vi "test_programm_webcam.vi"() -> ()   [LabVIEW 2014]
uses:
  <vilib>/userdefined/High Color/IMAQdx.ctl
  <vilib>/vision/driver/NI_Vision_Acquisition_Software.lvlib
  <vilib>/vision/NI_Vision_Development_Module.lvlib
panel:
  in  "pattern2":bool
  in  "Pattern2 Farbe":u32(colorbox)=16711680
  in  "x":i32
  in  "y":i32
  out "Pattern1 2":T1(plugin-control)
  in  "Template File Path (Pattern Matching 2)":path=path "C:/Users/Kroll/Desktop/Test_04012016/Pattern/pattern_1412.png"
  out "date/time string":string
  in  "file path (dialog if empty)":path=path "I:/123.txt"
  in  "Länge der Spur":i32=50
  out "Pattern1":T1(plugin-control)
  in  "Template File Path (Pattern Matching 1)":path=path "C:/Users/Kroll/Desktop/Test_04012016/Pattern/pattern_1412.png"
  out "Image 2":T1(plugin-control)
  in  "Programm anhalten":bool
  in  "Parameters Pattern":T2={"Number of Matches Requested"=1, "Minimum Match Score"=800.0, "Angle Ranges"=[{"Start Angle"=-180.0, "End Angle"=180.0}, {"Start Angle"=0.0, "End Angle"=360.0}]}
  in  "Mittelpunktgröße":sgl
  in  "millisecond multiple":u32
  out "Processed Frames/s":dbl
  in  "Länge des Pfeils":sgl=80.0
  out "Acquired Frames/s":dbl
  in  "pattern1":bool
  in  "Pattern1 Farbe":u32(colorbox)=16711680
  in  "x":i32
  in  "y":i32
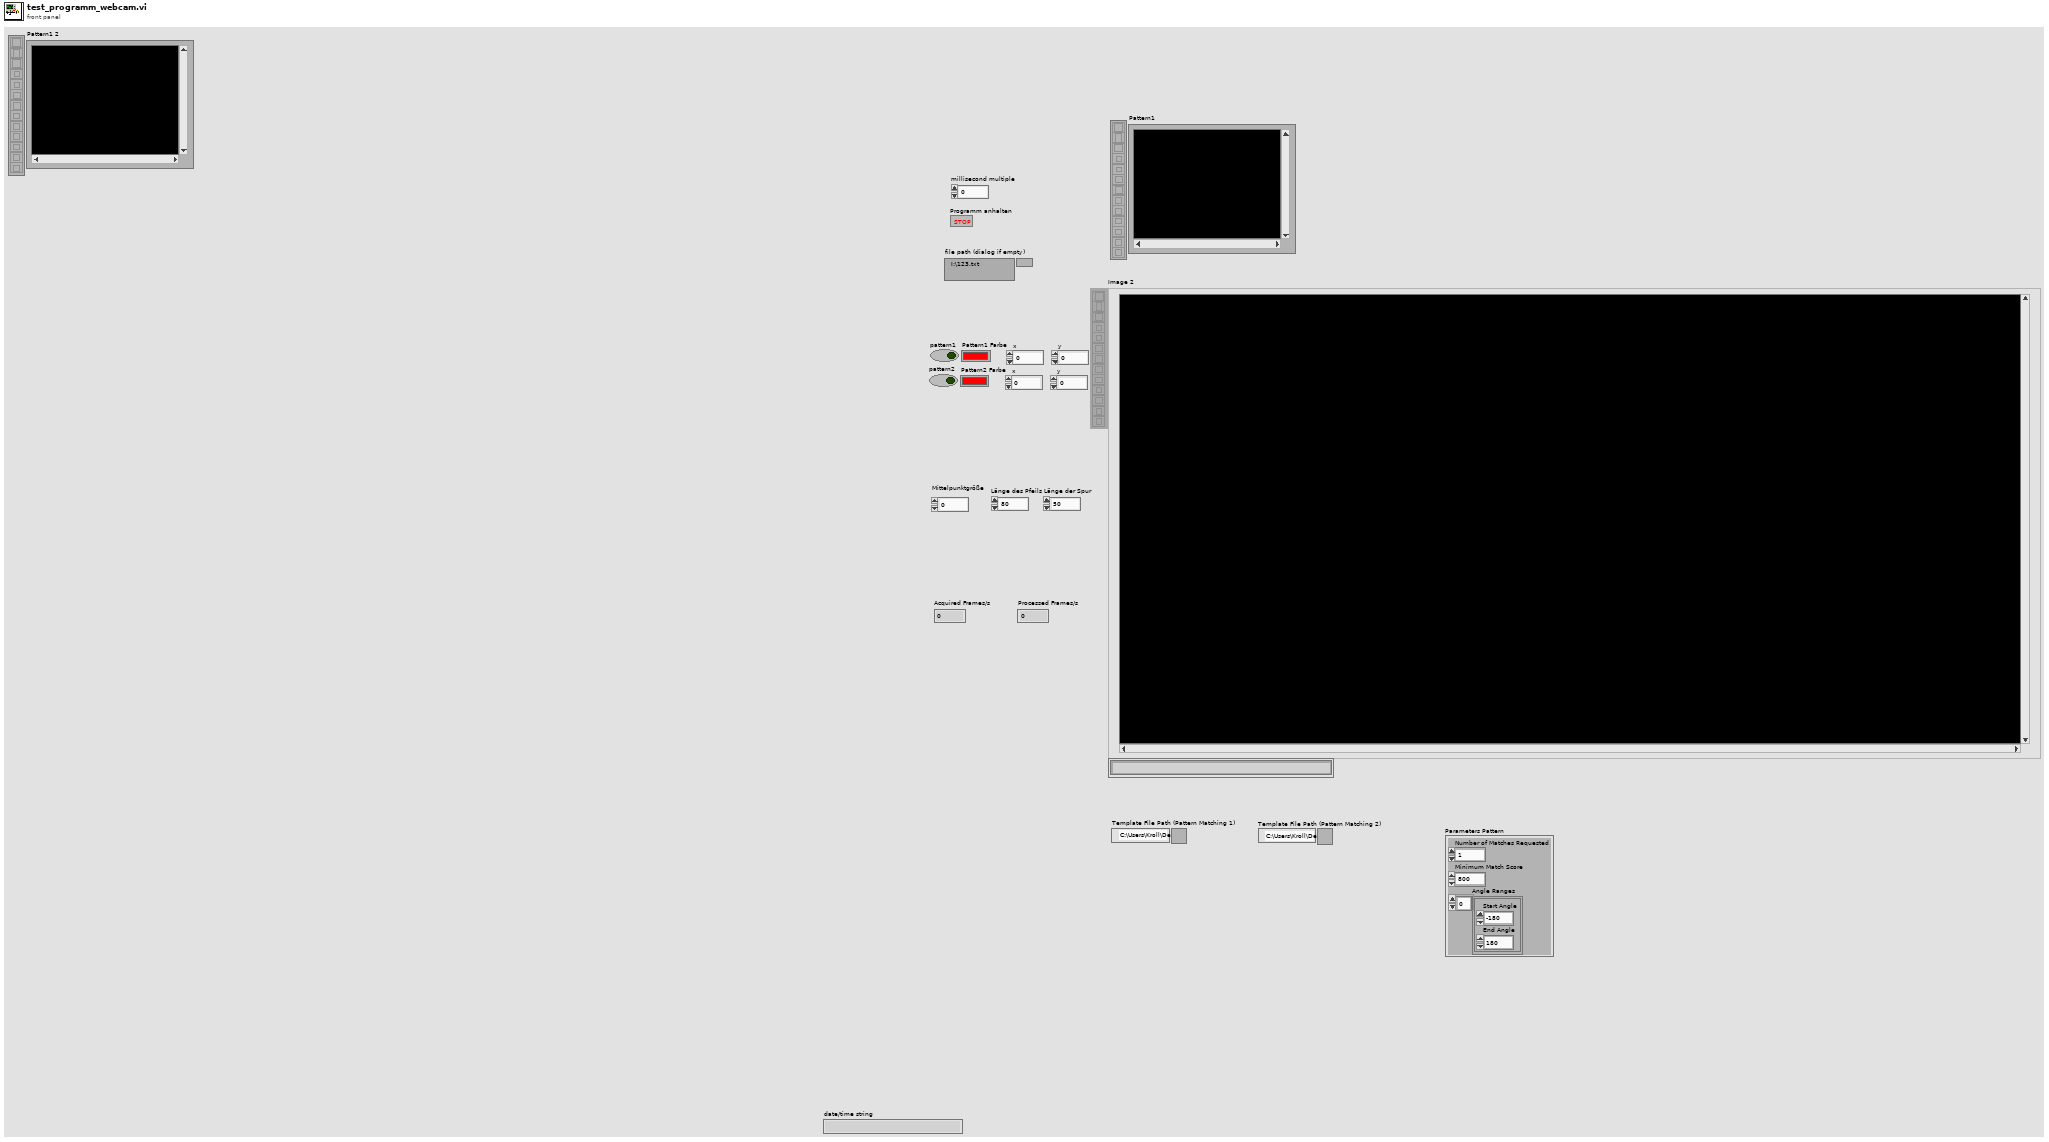
[diagram p1: front panel]
types:
  T1 = typedef "IMAQ Image.ctl" = refnum<image>
  T2 = cluster{"Number of Matches Requested":i32, "Minimum Match Score":sgl, "Angle Ranges":cluster{"Start Angle":sgl, "End Angle":sgl}[]}
  T3 = cluster{"Number of Histogram Bins":i32, "Blending Parameter (%)":dbl, "Maximum Iterations":i32}
  T4 = typedef "Image Type" = u32
  T5 = enum16{"open", "replace", "create", "open or create", "replace or create", "replace or create with confirmation"}
  T6 = typedef "IMAQdx.ctl" = refnum<k21>
  T7 = typedef "IMAQ Object Tracking Session.ctl" = refnum<k20>
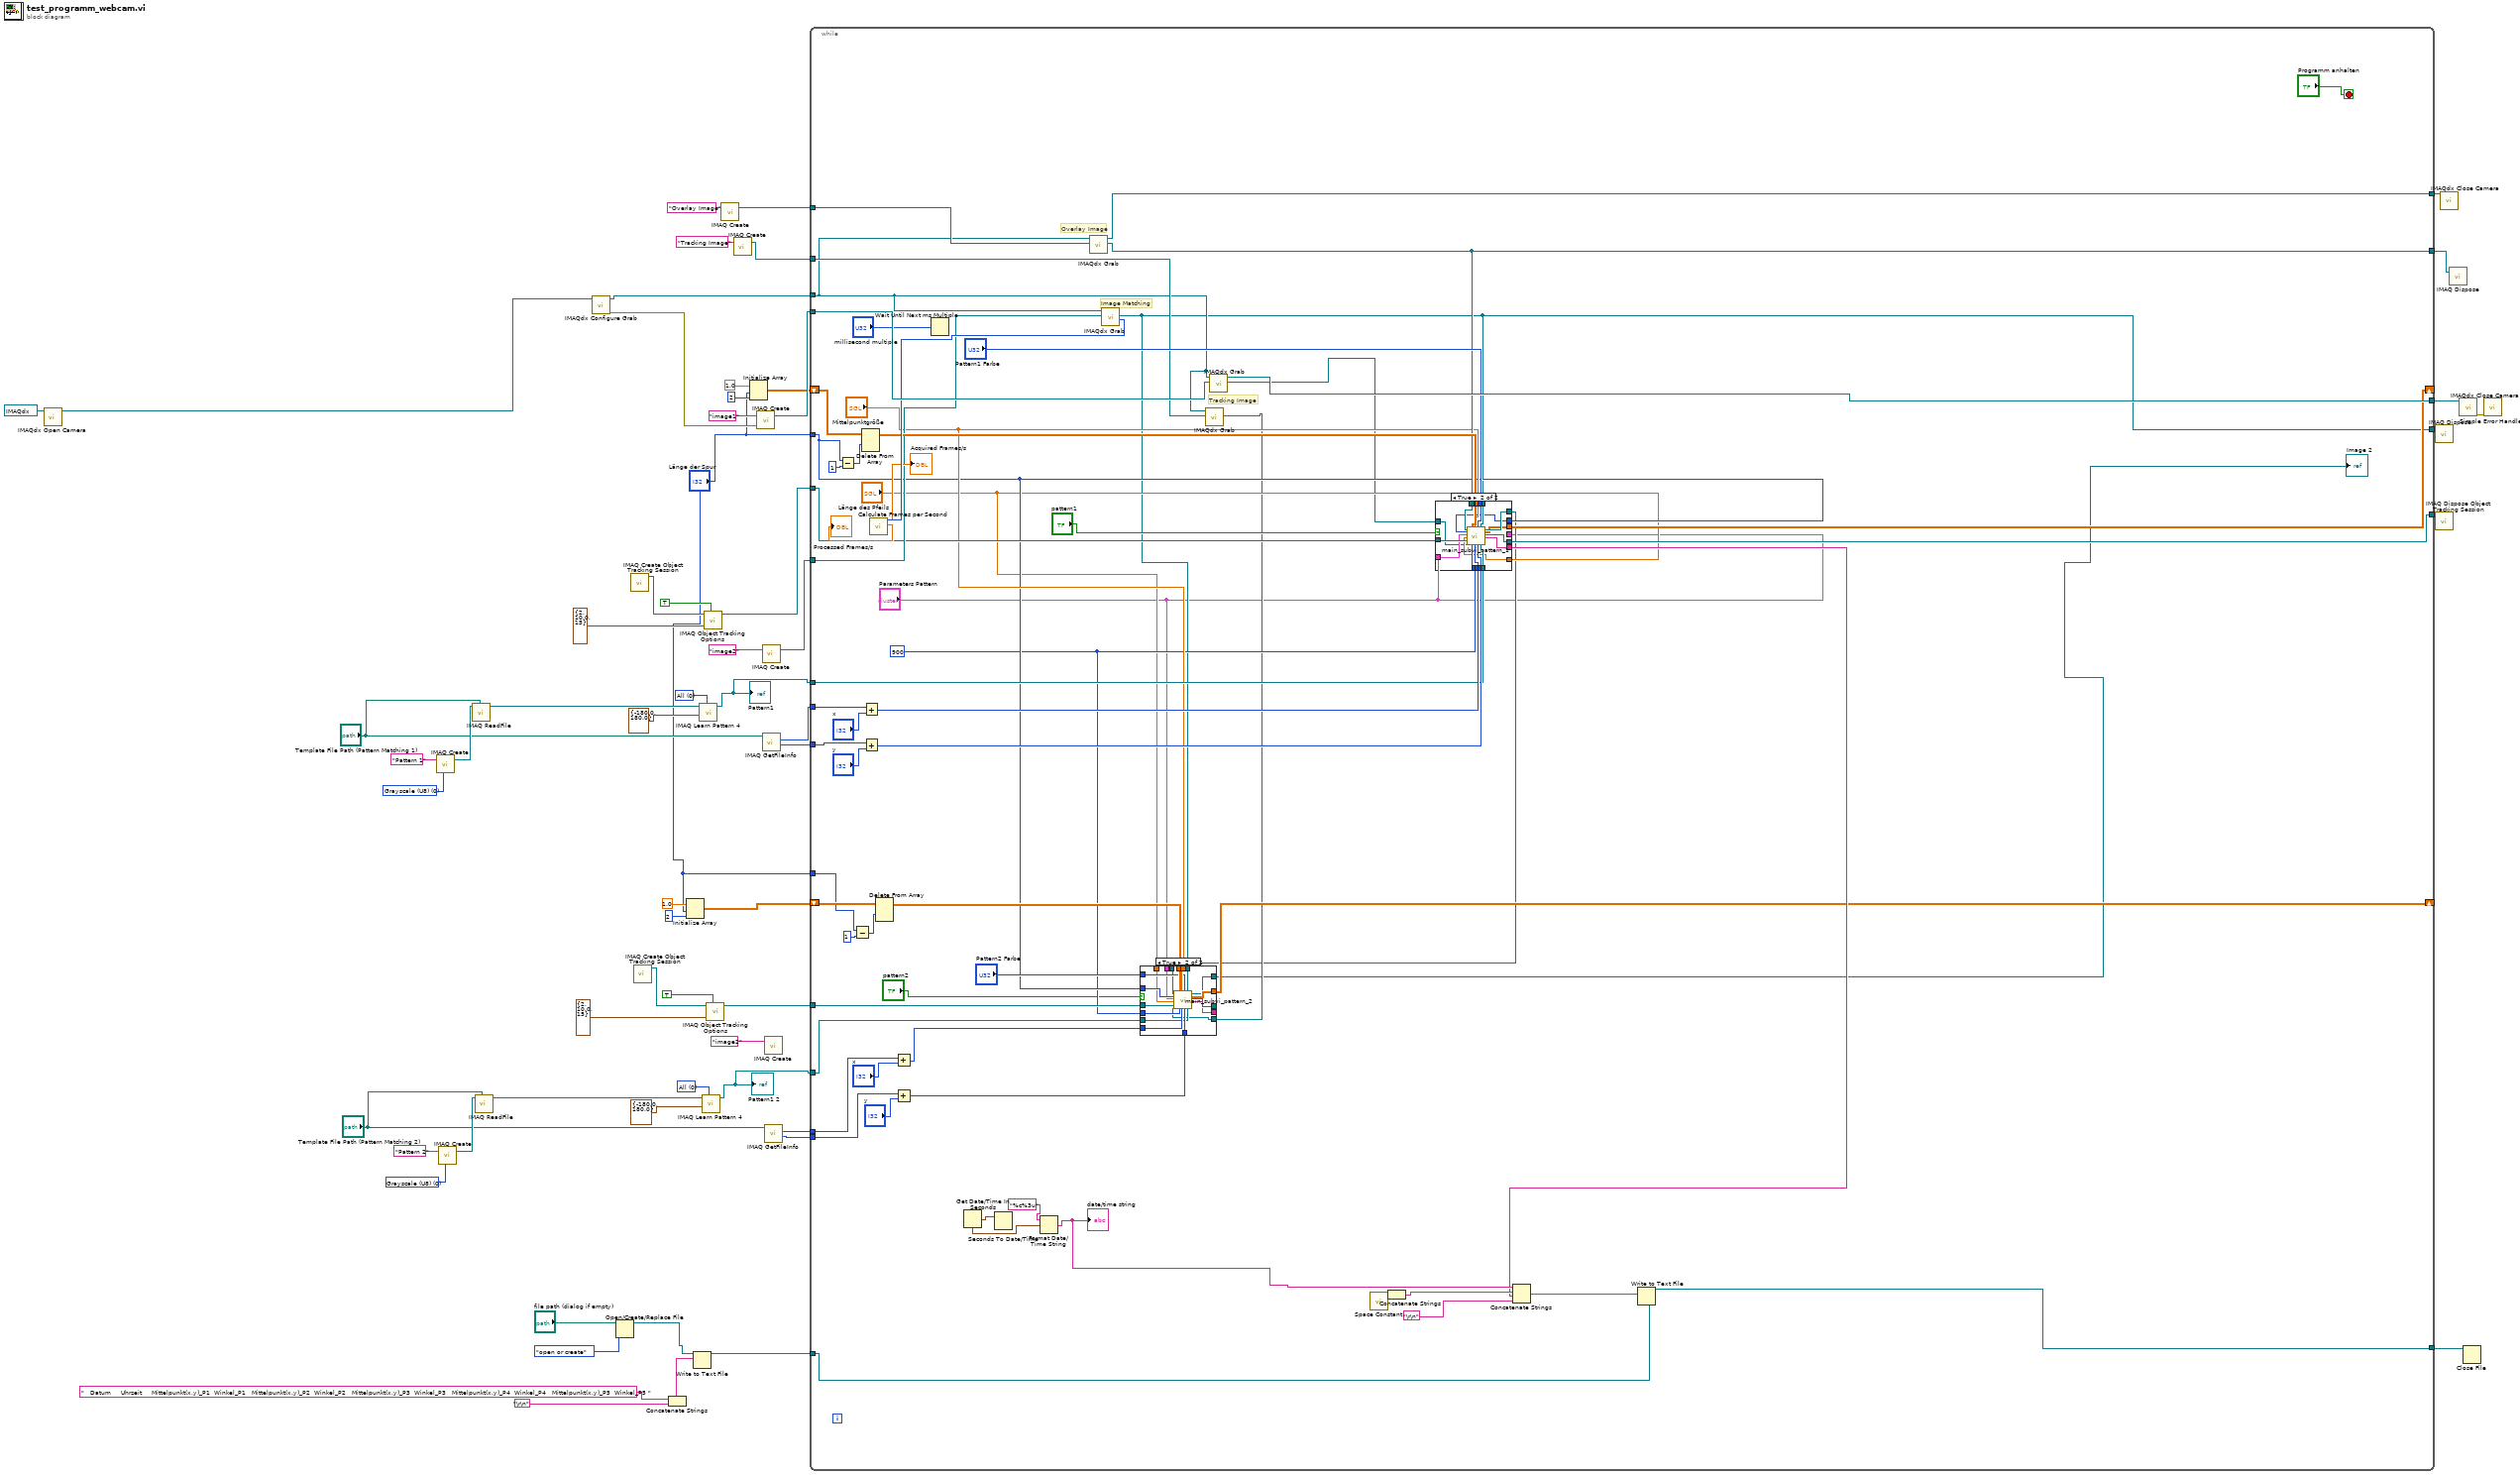
[diagram p0: block diagram]
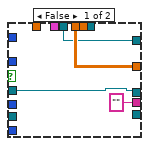
[diagram p2: hidden frame]
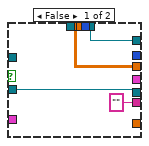
[diagram p3: hidden frame]
diagram:
  w16 = T4 0 items=["Grayscale (U8)", "Grayscale (I16)", "Grayscale (SGL)", "Complex (CSG)", "RGB (U32)", "HSL (U32)", "RGB (U64)", "Grayscale (U16)"] ("Image Type")
  w20 = 0 items=["All", "Low Discrepancy Sampling", "Grayscale Value Pyramid", "Gradients Pyramid"] ("Algorithm")
  w44 = T4 0 items=["Grayscale (U8)", "Grayscale (I16)", "Grayscale (SGL)", "Complex (CSG)", "RGB (U32)", "HSL (U32)", "RGB (U64)", "Grayscale (U16)"] ("Image Type")
  w48 = 0 items=["All", "Low Discrepancy Sampling", "Grayscale Value Pyramid", "Gradients Pyramid"] ("Algorithm")
  n1 = call <vilib>:"IMAQdx Open Camera.vi"("Session In"=T6 "cam4") -> ("Session Out"=w31:T6)  [unwired: 9 in, 1 out]
  n2 = call "IMAQ Create"("Image Name"="Pattern 1", "Image Type"=w44) -> ("New Image"=w45:T1)  [unwired: 3 in, 1 out]
  n3 = call "IMAQ Create"("Image Name"="Pattern 2", "Image Type"=w16) -> ("New Image"=w17:T1)  [unwired: 3 in, 1 out]
  n4 = call "IMAQ ReadFile"("File Path"="Template File Path (Pattern Matching 1)", "Image"=w45) -> ("Image Out"=w41:T1)  [unwired: 5 in, 4 out]
  n5 = call "IMAQ ReadFile"("File Path"="Template File Path (Pattern Matching 2)", "Image"=w17) -> ("Image Out"=w14:T1)  [unwired: 5 in, 4 out]
  n6 = call <vilib>:"IMAQdx Configure Grab.vi"("Session In"=w31) -> ("error out"=w62:errorcluster, "Session Out"=w60:T6)  [unwired: 9 in]
  n7 = Open/Create/Replace File(file path (use dialog)="file path (dialog if empty)", operation (0:open)=T5."open or create") -> (refnum out=w28:refnum<file>)  [unwired: 4 in, 2 out]
  n8 = call "IMAQ Create Object Tracking Session"() -> ("Object Tracking Session"=w40:T7)  [unwired: 1 in, 10 out]
  n9 = call "IMAQ Create Object Tracking Session"() -> ("Object Tracking Session"=w13:T7)  [unwired: 1 in, 10 out]
  n10 = Concatenate Strings("   Datum     Uhrzeit     Mittelpunkt(x,y)_P1  Winkel_P1   Mittelpunkt(x,y)_P2  Winkel_P2   Mittelpunkt(x,y)_P3  Winkel_P3   Mittelpunkt(x,y)_P4  Winkel_P4   Mittelpunkt(x,y)_P5  Winkel_P5 " ("string"), "\r\n") -> (w26:string)
  n11 = Initialize Array "Initialize Array"(1.0 ("element"), "Länge der Spur", 2 ("dimension size")) -> (w4:dbl[][])
  n12 = Write to Text File(file (use dialog)=w28, text=w26) -> (refnum out=w24:refnum<file>)  [unwired: 2 in, 2 out]
  n13 = call "IMAQ Learn Pattern 4"("Algorithm"=w48, "Angle Range"=cluster{"Start Angle":sgl, "End Angle":sgl} {"Start Angle"=-180.0, "End Angle"=180.0}, "Image"=w41) -> ("Template Image Out"=w42:T1)  [unwired: 6 in, 2 out]
  "Pattern1" <- w42
  n14 = call "IMAQ Learn Pattern 4"("Algorithm"=w20, "Angle Range"=cluster{"Start Angle":sgl, "End Angle":sgl} {"Start Angle"=-180.0, "End Angle"=180.0}, "Image"=w14) -> ("Template Image Out"=w9:T1)  [unwired: 6 in, 2 out]
  "Pattern1 2" <- w9
  n15 = call-poly "IMAQ Object Tracking Options"("Get/Set (Get)"=TRUE, "Mean Shift Options in"=T3 {"Number of Histogram Bins"=2, "Blending Parameter (%)"=10.0, "Maximum Iterations"=15}, "Object Tracking Session In"=w40) -> ("Object Tracking Session Out"=w39:T7)  [unwired: 6 in, 2 out]
  n16 = call-poly "IMAQ Object Tracking Options"("Get/Set (Get)"=TRUE, "Mean Shift Options in"=T3 {"Number of Histogram Bins"=2, "Blending Parameter (%)"=10.0, "Maximum Iterations"=15}, "Object Tracking Session In"=w13) -> ("Object Tracking Session Out"=w10:T7)  [unwired: 6 in, 2 out]
  n17 = call "IMAQ Create"("Image Name"="Overlay Image") -> ("New Image"=w35:T1)  [unwired: 4 in, 1 out]
  n18 = call "IMAQ Create"("Image Name"="Tracking Image") -> ("New Image"=w1:T1)  [unwired: 4 in, 1 out]
  n19 = Initialize Array "Initialize Array"(1.0 ("element"), "Länge der Spur", 2 ("dimension size")) -> (w50:dbl[][])
  n20 = call "IMAQ Create"("Image Name"="image1", "error in (no error)"=w62) -> ("New Image"=w59:T1)  [unwired: 3 in, 1 out]
  n21 = call "IMAQ Create"("Image Name"="image2") -> ("New Image"=w55:T1)  [unwired: 4 in, 1 out]
  n22 = call "IMAQ GetFileInfo"("File Path"="Template File Path (Pattern Matching 1)") -> ("Y Resolution"=w52:i32, "X Resolution"=w53:i32)  [unwired: 4 in, 5 out]
  n23 = call "IMAQ Create"("Image Name"="image2") -> ()  [unwired: 4 in, 2 out]
  n24 = call "IMAQ GetFileInfo"("File Path"="Template File Path (Pattern Matching 2)") -> ("Y Resolution"=w7:i32, "X Resolution"=w8:i32)  [unwired: 4 in, 5 out]
  n25 = while {
    tunnel: w60 -> [w68]
    tunnel: w59 -> [w126]
    tunnel: [w127] -> w57
    tunnel: [w64] -> w54
    tunnel: w55 -> [w112]
    tunnel: w53 -> [w113]
    tunnel: w52 -> [w114]
    shift-right: [w105] -> _
    shift-left: w50 -> [w121]
    tunnel: "Länge der Spur" -> [w80]
    tunnel: w42 -> [w102]
    tunnel: w39 -> [w106]
    tunnel: [w111] -> w37
    tunnel: w35 -> [w108]
    tunnel: [w103] -> w34
    tunnel: [w107] -> w33
    tunnel: w24 -> [w99]
    tunnel: [w95] -> w23
    tunnel: w10 -> [w79]
    tunnel: w9 -> [w75]
    tunnel: w8 -> [w90]
    tunnel: w7 -> [w89]
    shift-right: [w83] -> _
    shift-left: w4 -> [w86]
    tunnel: "Länge der Spur" -> [w85]
    tunnel: w1 -> [w69]
    stop <- "Programm anhalten" stop-if-true
    w78 = 900 ("Minimum Score")
    # "Overlay Image"
    # "Image Matching"
    # "Tracking Image"
    n26 = Subtract(x=w80, y=1) -> (x-y=w118:i32)
    n27 = Subtract(x=w85, y=1) -> (x-y=w87:i32)
    n28 = Delete From Array "Delete From Array"(array=w121, index (row)=w118) -> (array with subset deleted=w120:dbl[][])  [unwired: 2 in, 1 out]
    n29 = Add(x=w113, y="x") -> (x+y=w110:i32)
    n30 = Add(x=w114, y="y") -> (x+y=w109:i32)
    n31 = Delete From Array "Delete From Array"(array=w86, index (row)=w87) -> (array with subset deleted=w84:dbl[][])  [unwired: 2 in, 1 out]
    n32 = Add(x=w90, y="x") -> (x+y=w76:i32)
    n33 = Add(x=w89, y="y") -> (x+y=w77:i32)
    n34 = Wait Until Next ms Multiple(millisecond multiple="millisecond multiple") -> ()  [unwired: 1 out]
    n35 = Get Date/Time In Seconds() -> (seconds since 1Jan1904=w98:timestamp)
    n36 = Seconds To Date/Time(time stamp (now)=w98) -> ()  [unwired: 1 in, 1 out]
    n37 = Format Date/Time String(time format string (%c)="%c%3u", seconds (now)=w98) -> (date/time string=w96:string)  [unwired: 1 in]
    "date/time string" <- w96
    n38 = call <vilib>:"IMAQdx Grab.vi"("Image In"=w108, "Session In"=w68) -> ("Image Out"=w103:T1, "Session Out"=w107:T6)  [unwired: 6 in, 2 out]
    n39 = call <vilib>:"IMAQdx Grab.vi"("Image In"=w112, "Session In"=w68) -> ("Buffer Number Out"=w124:u32, "Image Out"=w64:T1)  [unwired: 6 in, 2 out]
    n40 = call <vilib>:"Calculate Frames per Second.vi"("Buffer Number"=w124) -> ("Processed Frames/s"=→"Processed Frames/s":dbl, "Acquired Frames/s"=→"Acquired Frames/s":dbl)  [unwired: 8 in, 1 out]
    n41 = call <vilib>:"IMAQdx Grab.vi"("Image In"=w69, "Session In"=w68) -> ("Image Out"=w67:T1)  [unwired: 6 in, 3 out]
    n42 = call <vilib>:"IMAQdx Grab.vi"("Image In"=w126, "Session In"=w68) -> ("Image Out"=w73:T1, "Session Out"=w127:T6)  [unwired: 6 in, 2 out]
    n43 = call <vilib>:"Space Constant.vi"() -> ("String"=w101:string)
    n44 = Concatenate Strings(w101, w101) -> (w94:string)
    n45 = case shown="True" "pattern1" {
      tunnel: w120 -> [w151 w162]
      tunnel: "Länge des Pfeils" -> [_ w157]
      tunnel: "Mittelpunktgröße" -> [_ w161]
      tunnel: w78 -> [_ w164]
      tunnel: [w152 w169] -> w111
      tunnel: w110 -> [_ w165]
      tunnel: w109 -> [_ w166]
      tunnel: w64 -> [w153 w160]
      tunnel: w106 -> [w152 w163]
      tunnel: w80 -> [_ w154]
      tunnel: [w151 w170] -> w105
      tunnel: "Pattern1 Farbe" -> [_ w155]
      tunnel: w103 -> [_ w159]
      tunnel: w102 -> [_ w167]
      tunnel: ["" ("String") w168] -> w92
      tunnel: "Parameters Pattern" -> [_ _]
      tunnel: [w153 w171] -> w65
      tunnel: w73 -> [_ w156]
      tunnel: "Parameters Pattern" -> [_ w158]
      frame False {
      }
      frame True {
        n46 = call "main_subvi_pattern_1.vi"("Refnum Original Bild"=w159, "Länge der Spur"=w154, "Parameters Pattern"=w158, "Länge des Pfeils"=w157, "Object Tracking Session Out in"=w163, "Refnum Tracking"=w156, "Array in"=w162, "Minimum Score"=w164, "Mittelpunktgröße"=w161, "Numeric 2"=w165, "Pattern1 Farbe"=w155, "Numeric"=w166, "Image Matching"=w160, "Template Image In"=w167) -> ("Refnum OUt"=w171:T1, "Array out"=w170:dbl[][], "Object Tracking Session Out out"=w169:T7, "String"=w168:string)  [unwired: 2 in]
      }
    }
    n47 = case shown="True" "pattern2" {
      tunnel: [w129 w149] -> _
      tunnel: [w130 w148] -> w83
      tunnel: ["" ("String") w147] -> _
      tunnel: [w128 w146] -> w66
      tunnel: w84 -> [w130 w145]
      tunnel: w64 -> [_ w144]
      tunnel: "Mittelpunktgröße" -> [_ w143]
      tunnel: "Pattern2 Farbe" -> [_ w142]
      tunnel: w80 -> [_ w141]
      tunnel: w79 -> [w129 w140]
      tunnel: w65 -> [w128 w139]
      tunnel: "Parameters Pattern" -> [_ w138]
      tunnel: w78 -> [_ w137]
      tunnel: w77 -> [_ w136]
      tunnel: w76 -> [_ w135]
      tunnel: w75 -> [_ w134]
      tunnel: "Länge des Pfeils" -> [_ w133]
      tunnel: w67 -> [_ w132]
      frame False {
      }
      frame True {
        n48 = call "main_subvi_pattern_2.vi"("Refnum Original Bild"=w139, "Länge der Spur"=w141, "Parameters Pattern"=w138, "Länge des Pfeils"=w133, "Object Tracking Session Out in"=w140, "Refnum Tracking"=w132, "Array in"=w145, "Minimum Score"=w137, "Mittelpunktgröße"=w143, "Numeric 2"=w135, "Pattern1 Farbe"=w142, "Numeric"=w136, "Image Matching"=w144, "Template Image In"=w134) -> ("Refnum OUt"=w146:T1, "Array out"=w148:dbl[][], "Object Tracking Session Out out"=w149:T7, "String"=w147:string)  [unwired: 2 in]
      }
    }
    "Image 2" <- w66
    n49 = Concatenate Strings(w96, w94, w92, "\r\n") -> (w100:string)
    n50 = Write to Text File(file (use dialog)=w99, text=w100) -> (refnum out=w95:refnum<file>)  [unwired: 2 in, 2 out]
  }
  n51 = call "IMAQ Dispose"("Image"=w54) -> ()  [unwired: 5 in, 1 out]
  n52 = call "IMAQ Dispose Object Tracking Session"("Object Tracking Session"=w37) -> ()  [unwired: 1 in, 10 out]
  n53 = call <vilib>:"IMAQdx Close Camera.vi"("Session In"=w33) -> ()  [unwired: 10 in, 1 out]
  n54 = call "IMAQ Dispose"("Image"=w34) -> ()  [unwired: 5 in, 1 out]
  n55 = call <vilib>:"IMAQdx Close Camera.vi"("Session In"=w57) -> ("error out"=w58:errorcluster)  [unwired: 10 in]
  n56 = Close File(refnum=w23) -> ()  [unwired: 1 in, 2 out]
  n57 = call <vilib>:"Simple Error Handler.vi"("error in (no error)"=w58) -> ()  [unwired: 4 in, 5 out]
